vi "MSScript_Format_CLFreqScan.vi"(9 "ValueArray":string[](array[string]), 10 "TagArray":string[](array[string]), 11 "MSScript in":refnum<class "MSScript.lvclass">) -> (0 "ValueErrorArray":bool[](array[boolean]), 1 "TagErrorArray":bool[](array[boolean]), 2 "ParamErrorArray":bool[](array[boolean]), 3 "Data":variant, 4 "#ofParamError":bool, 6 "Warning?":bool)   [LabVIEW 2018, in "MSScript.lvclass"]
uses:
  MSScript.lvclass
  Ctl/MSEditorParam CLFreqScan.ctl
  MSScript_Transform_Extended.vi
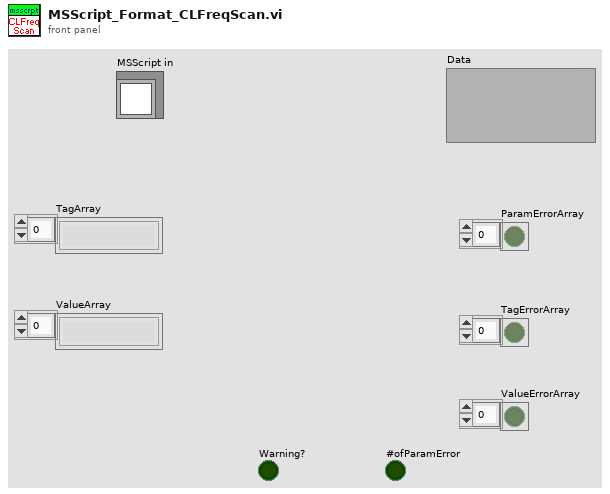
[diagram p1: front panel]
types:
  T1 = typedef "MSEditorParam CLFreqScan.ctl" = cluster{"targetfreq":ext, "time":ext}
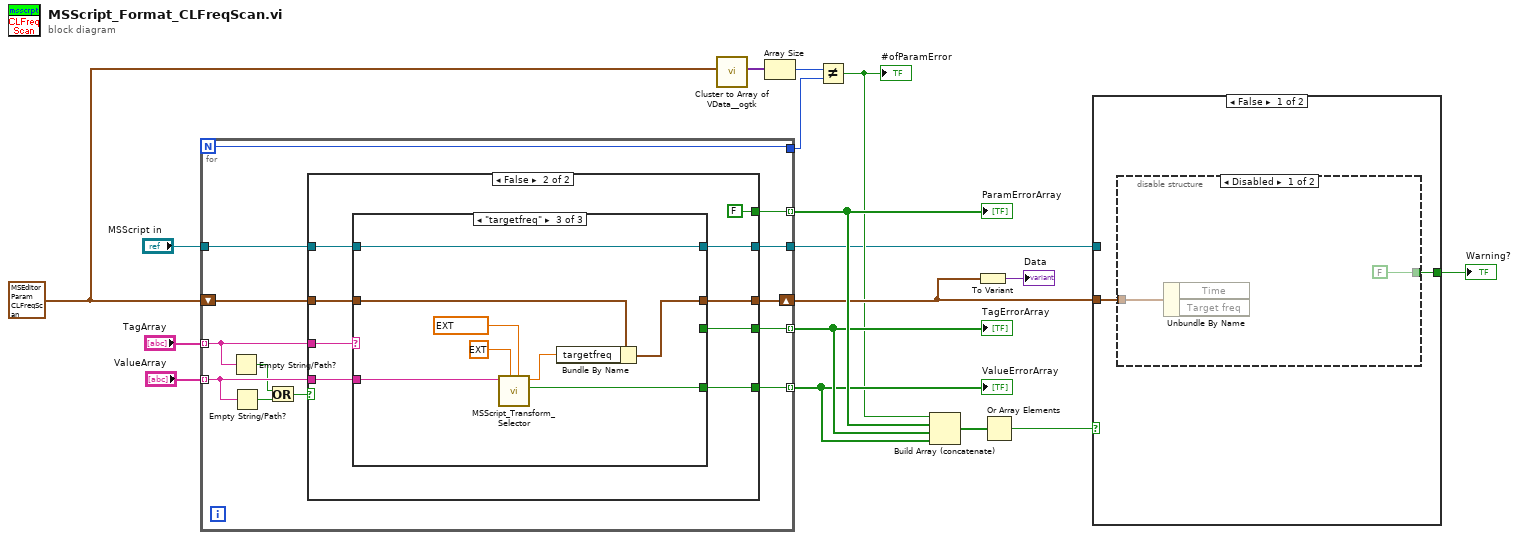
[diagram p0: block diagram]
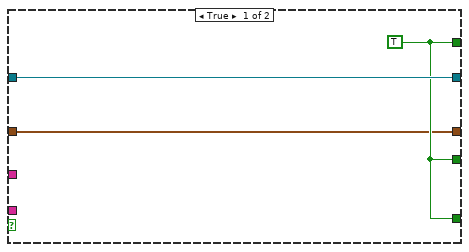
[diagram p4: hidden frame]
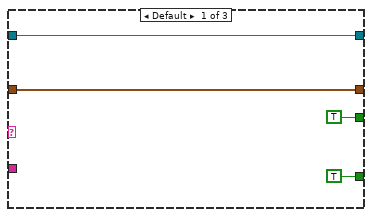
[diagram p5: hidden frame]
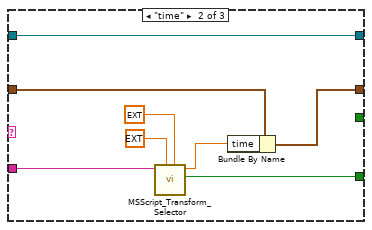
[diagram p6: hidden frame]
diagram:
  w2 = T1 {"targetfreq"=1.0, "time"=1.0} ("ParamValueType")
  n1 = for {
    N -> [w18]
    tunnel: "TagArray" -> [w26] mode=indexing
    tunnel: "ValueArray" -> [w25] mode=indexing
    tunnel: [w30] -> w9 mode=indexing
    tunnel: "MSScript in" -> [w29]
    tunnel: [w28] -> w8 mode=indexing
    tunnel: [w27] -> w3
    tunnel: [w21] -> w10 mode=indexing
    shift-right: [w19] -> w5
    shift-left: w2 -> [w20]
    tunnel: [w18] -> w12
    n2 = Empty String/Path?(string/path=w26) -> (empty?=w23:bool)
    n3 = Empty String/Path?(string/path=w25) -> (empty?=w24:bool)
    n4 = Or(x=w23, y=w24) -> (x .or. y?=w22:bool)
    n5 = case shown="False" w22 {
      tunnel: [w32 w35] -> w30
      tunnel: w29 -> [w33 w41]
      tunnel: [w32 w34] -> w28
      tunnel: [w33 w37] -> w27
      tunnel: w26 -> [_ w39]
      tunnel: w25 -> [_ w38]
      tunnel: [w32 FALSE] -> w21
      tunnel: w20 -> [w31 w40]
      tunnel: [w31 w36] -> w19
      frame True {
        w32 = TRUE
      }
      frame False {
        n6 = case shown="\"targetfreq\"" w39 {
          tunnel: [TRUE _ _] -> w35
          tunnel: w41 -> [w44 w52 w60]
          tunnel: w38 -> [_ w53 w61]
          tunnel: [TRUE ("Value Error?") w54 w62] -> w34
          tunnel: [w44 w52 w60] -> w37
          tunnel: w40 -> [w43 w50 w58]
          tunnel: [w43 w49 w57] -> w36
          frame Default {
          }
          frame "time" {
            n7 = call-poly "MSScript_Transform_Selector.vi"("upper limit (Inf)"=ext 60.0 ("upper limit"), "lower limit (-Inf)"=ext 0.0 ("lower limit"), "Check_Str"=w53) -> ("Value Error?"=w54:bool, "Value Output"=w51:ext)  [unwired: 6 in, 1 out]
            n8 = Bundle By Name(cluster=w50, "time"=w51) -> (w49:T1)
          }
          frame "targetfreq" {
            n9 = call-poly "MSScript_Transform_Selector.vi"("upper limit (Inf)"=ext 2000000.0 ("upper limit"), "lower limit (-Inf)"=ext 1.0 ("lower limit"), "Check_Str"=w61) -> ("Value Error?"=w62:bool, "Value Output"=w59:ext)  [unwired: 6 in, 1 out]
            n10 = Bundle By Name(cluster=w58, "targetfreq"=w59) -> (w57:T1)
          }
        }
      }
    }
  }
  "TagErrorArray" <- w9
  "ValueErrorArray" <- w8
  "ParamErrorArray" <- w10
  n11 = call <userlib>:"Cluster to Array of VData__ogtk.vi"("Cluster"=w2) -> ("Array of VData"=w14:variant[])  [unwired: 9 in, 1 out]
  n12 = Array Size(array=w14) -> (size(s)=w13:i32)
  n13 = Not Equal?(x=w13, y=w12) -> (x != y?=w4:bool)
  "#ofParamError" <- w4
  n14 = Build Array (concatenate)(w4, w10, w9, w8) -> (w7:bool[])
  n15 = To Variant(anything=w5) -> (Variant=→"Data":variant)
  n16 = Or Array Elements(Boolean array=w7) -> (logical OR=w6:bool)
  n17 = case shown="False" w6 {
    tunnel: w5 -> [w64 _]
    tunnel: w3 -> [_ _]
    tunnel: [w63 _] -> w1
    frame False {
      n18 = disable-structure shown="Disabled" {
        disable-tunnel: w64 -> [w66 _]
        disable-tunnel: [FALSE _] -> w63
        frame Disabled {
          n19 = Unbundle By Name(w66) -> ()  [unwired: 2 out]
        }
        frame Enabled {
        }
      }
    }
    frame True {
    }
  }
  "Warning?" <- w1
